vi "RSZVB Set Font Size.vi"(8 "error in (no error)":errorcluster {"code" format="%.0x"}, 10 "Font Size (100 %)":i32=100, 11 "VISA session":refnum<visa-resource-name>) -> (0 "error out":errorcluster {"code" format="%.0x"}, 3 "dup VISA session":refnum<visa-resource-name>)   [LabVIEW 2011]
doc: "This VI defines the size of the fonts in the diagram on a relative scale. \n\nRemote-control command(s):\nDISPlay:RFSize"
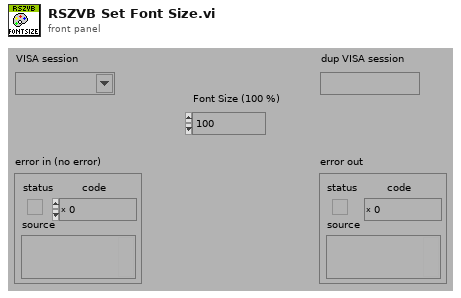
[diagram p1: front panel]
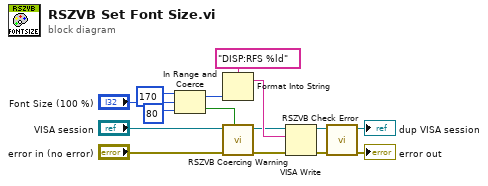
[diagram p0: block diagram]
diagram:
  n1 = In Range and Coerce(upper limit=170, x="Font Size (100 %)", lower limit=80) -> (coerced(x)=w3:i32, In Range?=w15:bool)
  n2 = Format Into String(format string="DISP:RFS %ld", w3) -> (resulting string=w14:string)  [unwired: 2 in, 1 out]
  n3 = call "RSZVB Coercing Warning.vi"("In Range?"=w15, "error in (no error)"="error in (no error)", "VISA session"="VISA session") -> ("error out"=w11:errorcluster, "dup VISA session"=w10:refnum<visa-resource-name>)  [unwired: 7 in]
  n4 = VISA Write(VISA resource name=w10, write buffer=w14, error in (no error)=w11) -> (VISA resource name out=w13:refnum<visa-resource-name>, error out=w12:errorcluster)  [unwired: 1 out]
  n5 = call "RSZVB Check Error.vi"("error in (no error)"=w12, "VISA session"=w13) -> ("error out"=→"error out":errorcluster, "dup VISA session"=→"dup VISA session":refnum<visa-resource-name>)  [unwired: 8 in]
